vi "Apply Stimulus.vi"(8 "error in (no error)":errorcluster, 10 "Acquisition Context":T1, 11 "Stimulus in":refnum<k21>) -> (0 "error out":errorcluster)   [LabVIEW 2026, in "Acquisition.lvlib"]
uses:
  Acquisition.lvlib
  <vilib>/DAQmx/write.llb/DAQmx Write (Analog DBL 1Chan 1Samp).vi
  Acquisition Context.ctl
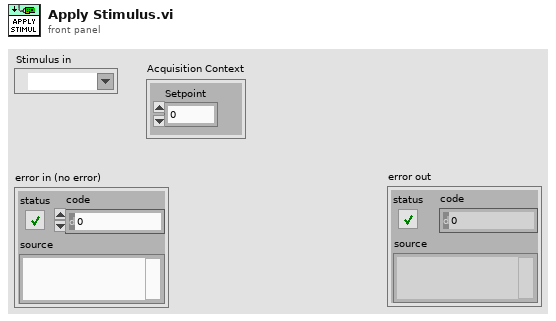
[diagram p1: front panel]
types:
  T1 = typedef "Acquisition Context.ctl" = cluster{"Setpoint":dbl}
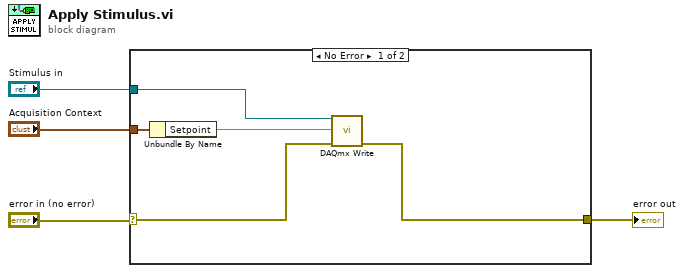
[diagram p0: block diagram]
diagram:
  n1 = case shown="No Error" "error in (no error)" {
    selector: "error in (no error)" -> [w6 w10]
    tunnel: "Acquisition Context" -> [w9 _]
    tunnel: "Stimulus in" -> [w7 _]
    tunnel: [w5 w10] -> w1
    frame No Error {
      n2 = Unbundle By Name(w9) -> ("Setpoint"=w8:dbl)
      n3 = call-poly <vilib>:"DAQmx Write.vi"("task/channels in"=w7, "data"=w8, "error in"=w6) -> ("error out"=w5:errorcluster)  [unwired: 10 in, 2 out]
    }
    frame Error {
    }
  }
  "error out" <- w1
